vi "Read Instrument Data.vi"(8 "error in (no error)":errorcluster, 9 "byte count":u32=256, 11 "VISA resource name":refnum<visa-resource-name>) -> (0 "error out":errorcluster, 1 "return byte count":u32, 2 "Read String":string, 3 "VISA resource name out":refnum<visa-resource-name>)   [LabVIEW 2010, in "Temptronic TP04300.lvlib"]
doc: "This VI reads data from the instrument's output buffer and returns it to the specified variable in memory.\n\nNotes:\n\n(1) Because the instrument may return both numeric and text data in response to queries this function returns the data in string format.\n\n(2) If valid data is not available at the instrument's output buffer when this function is called the instrument will hang up and the function will not return until it times out. If the time-out is disabled this function will hang indefinitely and it may be necessary to reboot the computer to break out."
uses:
  Temptronic TP04300.lvlib
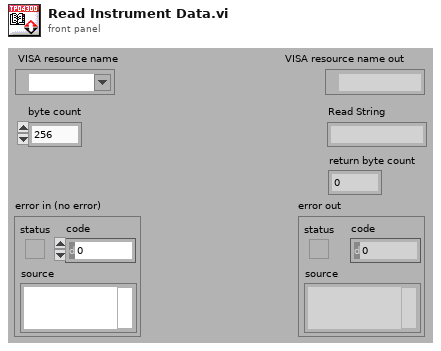
[diagram p1: front panel]
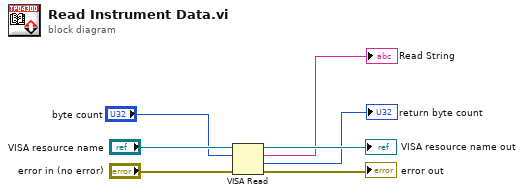
[diagram p0: block diagram]
diagram:
  n1 = VISA Read(VISA resource name="VISA resource name", byte count="byte count", error in (no error)="error in (no error)") -> (VISA resource name out=→"VISA resource name out":refnum<visa-resource-name>, read buffer=→"Read String":string, return count=→"return byte count":u32, error out=→"error out":errorcluster)
